vi "Set Cursor Busy.vi"(8 "error in (no error)":errorcluster, 10 "Disable Click?":bool, 11 "IViewManager In":refnum<class "IViewManager.lvclass">) -> (0 "error out":errorcluster, 3 "IViewManager Out":refnum<class "IViewManager.lvclass">)   [LabVIEW 2020, in "IViewManager.lvlib" / "IViewManager.lvclass"]
doc: "<License>\nCopyright © 2017 Composed Systems, LLC | All rights reserved\nwww.composed.io\n\nAuthor: Ethan Stern <ethan.stern@composed.io>\n\nThis software is provided \"AS IS\" WITHOUT WARRANTIES, either express or implied, AND IS FOR EDUCATIONAL PURPOSES ONLY.\n</License>"
uses:
  <vilib>/gpm_packages/@cs/mva-viewable/Source/IViewManager/IViewManager/IViewManager.lvclass
  <vilib>/gpm_packages/@cs/mva-viewable/Source/IViewManager/IViewManager/IViewManager.lvclass/IViewManager.ctl
  <vilib>/gpm_packages/@cs/mva-viewable/Source/IViewable/IViewable Messages/Set Cursor Busy Msg/Set Cursor Busy Msg.lvclass/Set Cursor Busy Msg.ctl
  <vilib>/ActorFramework/Message Enqueuer/Message Enqueuer.lvclass/Message Enqueuer.ctl
  <vilib>/ActorFramework/Message Enqueuer/Enqueue.vi
  <vilib>/gpm_packages/@cs/mva-viewable/Source/IViewable/IViewable Messages/Set Cursor Busy Msg/Set Cursor Busy Msg.lvclass
  C:/Program Files/National Instruments/LabVIEW 2020/vi.lib/ActorFramework/Message/Message.lvclass
  <vilib>/ActorFramework/Message Priority Queue/Priority Enqueue.vi
  <vilib>/gpm_packages/@cs/mva-viewable/Source/IViewable/IViewable/IViewable.lvclass
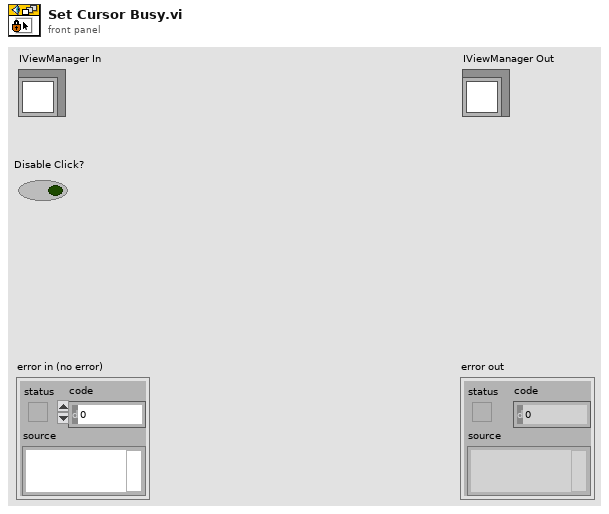
[diagram p1: front panel]
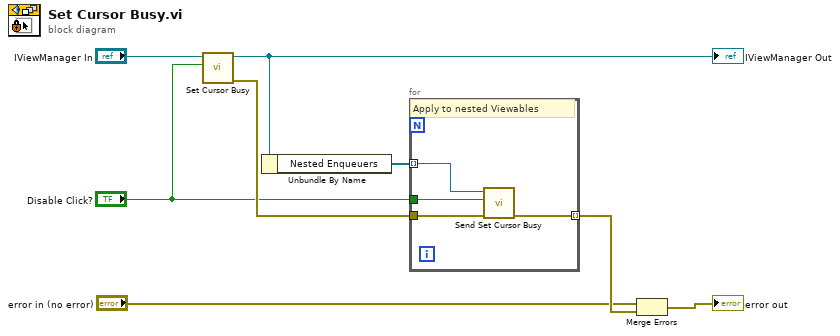
[diagram p0: block diagram]
diagram:
  n1 = call-parent "Set Cursor Busy.vi"("Disable Click?"="Disable Click?", "IViewable In"="IViewManager In") -> ("error out"=w8:errorcluster, "IViewable Out"=w6:refnum<class "IViewManager.lvclass">)  [unwired: 8 in]
  "IViewManager Out" <- w6
  n2 = Unbundle By Name(w6) -> ("Nested Enqueuers"=w4:refnum<class "Message Enqueuer.lvclass">[])
  n3 = for {
    tunnel: w4 -> [w12] mode=indexing
    tunnel: "Disable Click?" -> [w9]
    tunnel: w8 -> [w11]
    tunnel: [w10] -> w7 mode=indexing
    # "Apply to nested Viewables"
    n4 = call <vilib>:"Send Set Cursor Busy.vi"("error in (no error)"=w11, "Disable Click?"=w9, "Message Enqueuer"=w12) -> ("error out"=w10:errorcluster)  [unwired: 7 in, 1 out]
  }
  n5 = Merge Errors("error in (no error)", w7) -> (→"error out":errorcluster)
